vi "Frame_to_word_15693.vi"() -> ()   [LabVIEW 2019]
uses:
  <vilib>/addons/Modulation/Analog/support/mod_Set Error Source.vi
  <vilib>/addons/Modulation/Digital/Support/Common/Validators/mod_Generate Filter Coefficients Validate.vi
  <vilib>/addons/Modulation/Digital/General/subVIs/mod_Generate Filter Coefficients.vi
  <vilib>/addons/Modulation/Digital/General/MT Generate ASK system parameters (M).vi
  <vilib>/addons/Modulation/Analog/MT Modulate AM (DSB).vi
  <vilib>/addons/Modulation/Analog/MT Upconvert Baseband (Real).vi
  <vilib>/measure/macond.llb/IIR Filter for 1 Chan.vi
  <vilib>/express/express analysis/Spectral/Block/exnSpectralBlock spectral measurements RMS poly.vi
  <vilib>/express/express analysis/Spectral/Block/exnSpectralBlock spectral measurements RMS WFM.vi
  <vilib>/addons/Modulation/Analog/MT Downconvert Passband (Real).vi
  <vilib>/addons/Modulation/Analog/MT Demodulate AM (DSB).vi
  <vilib>/ErrorRing/Error Ring.xnode
  <vilib>/express/express analysis/Spectral/XNode/ExpressSpectralMeasurementsBlockNode.xnode
  <vilib>/addons/Modulation/niAMT.lvlib
  <vilib>/measure/NI_MAPro.lvlib
  <vilib>/addons/Modulation/niDMT.lvlib
panel:
  out "lo(x)":u8 format="%x"
  out "hi(x)":u8 format="%x"
  out "DEMODulate 2":cluster{"t0":dbl, "dt":dbl, "Y":dbl[]}(graph)
  out "Array of byte":u8[](array[numeric]) format="%x"
  out "decode":cluster{"t0":dbl, "dt":dbl, "Y":dbl[]}(graph)
  out "Command":cluster{"t0":dbl, "dt":dbl, "Y":dbl[]}(graph)
  out "DEMODulate":cluster{"t0":dbl, "dt":dbl, "Y":dbl[]}(graph)
  out "spectrum analog signal 6":waveform(dbl)(graph)
  out "spectrum analog signal 5":cluster{"t0":dbl, "dt":dbl, "Y":dbl[]}(graph)
  out "Analog signal 8":waveform(dbl)(graph)
  out "spectrum analog signal 4":cluster{"t0":dbl, "dt":dbl, "Y":dbl[]}(graph)
  out "antenna":waveform(dbl)(graph)
  out "summ":waveform(dbl)(graph)
  out "antenna 2":waveform(dbl)(graph)
  out "spectrum analog signal 3":cluster{"t0":dbl, "dt":dbl, "Y":dbl[]}(graph)
  out "spectrum analog signal 2":cluster{"t0":dbl, "dt":dbl, "Y":dbl[]}(graph)
  out "spectrum analog signal":cluster{"t0":dbl, "dt":dbl, "Y":dbl[]}(graph)
  out "SOF+DATA+EOF 2":cluster{"t0":dbl, "dt":dbl, "Y":dbl[]}(graph)
  in  "Value":u8[](array[numeric])=[50] format="%x"
  in  "Mask lenght":u8[](array[numeric])=[119] format="%x"
  in  "AFI":u8[](array[numeric])=[47] format="%x"
  in  "Inventory":u8[](array[numeric])=[161] format="%x"
  out "SOF+DATA+EOF":cluster{"t0":dbl, "dt":dbl, "Y":dbl[]}(graph)
  out "Video":cluster{"t0":dbl, "dt":dbl, "Y":dbl[]}(graph)
  out "video Miller":cluster{"t0":dbl, "dt":dbl, "Y":dbl[]}(graph)
  in  "CARRIER (hz)":dbl
  in  "BIT RATE":dbl
  out "100% ASK":waveform(dbl)(graph)
  in  "Flag":u8[](array[numeric])=[38] format="%x"
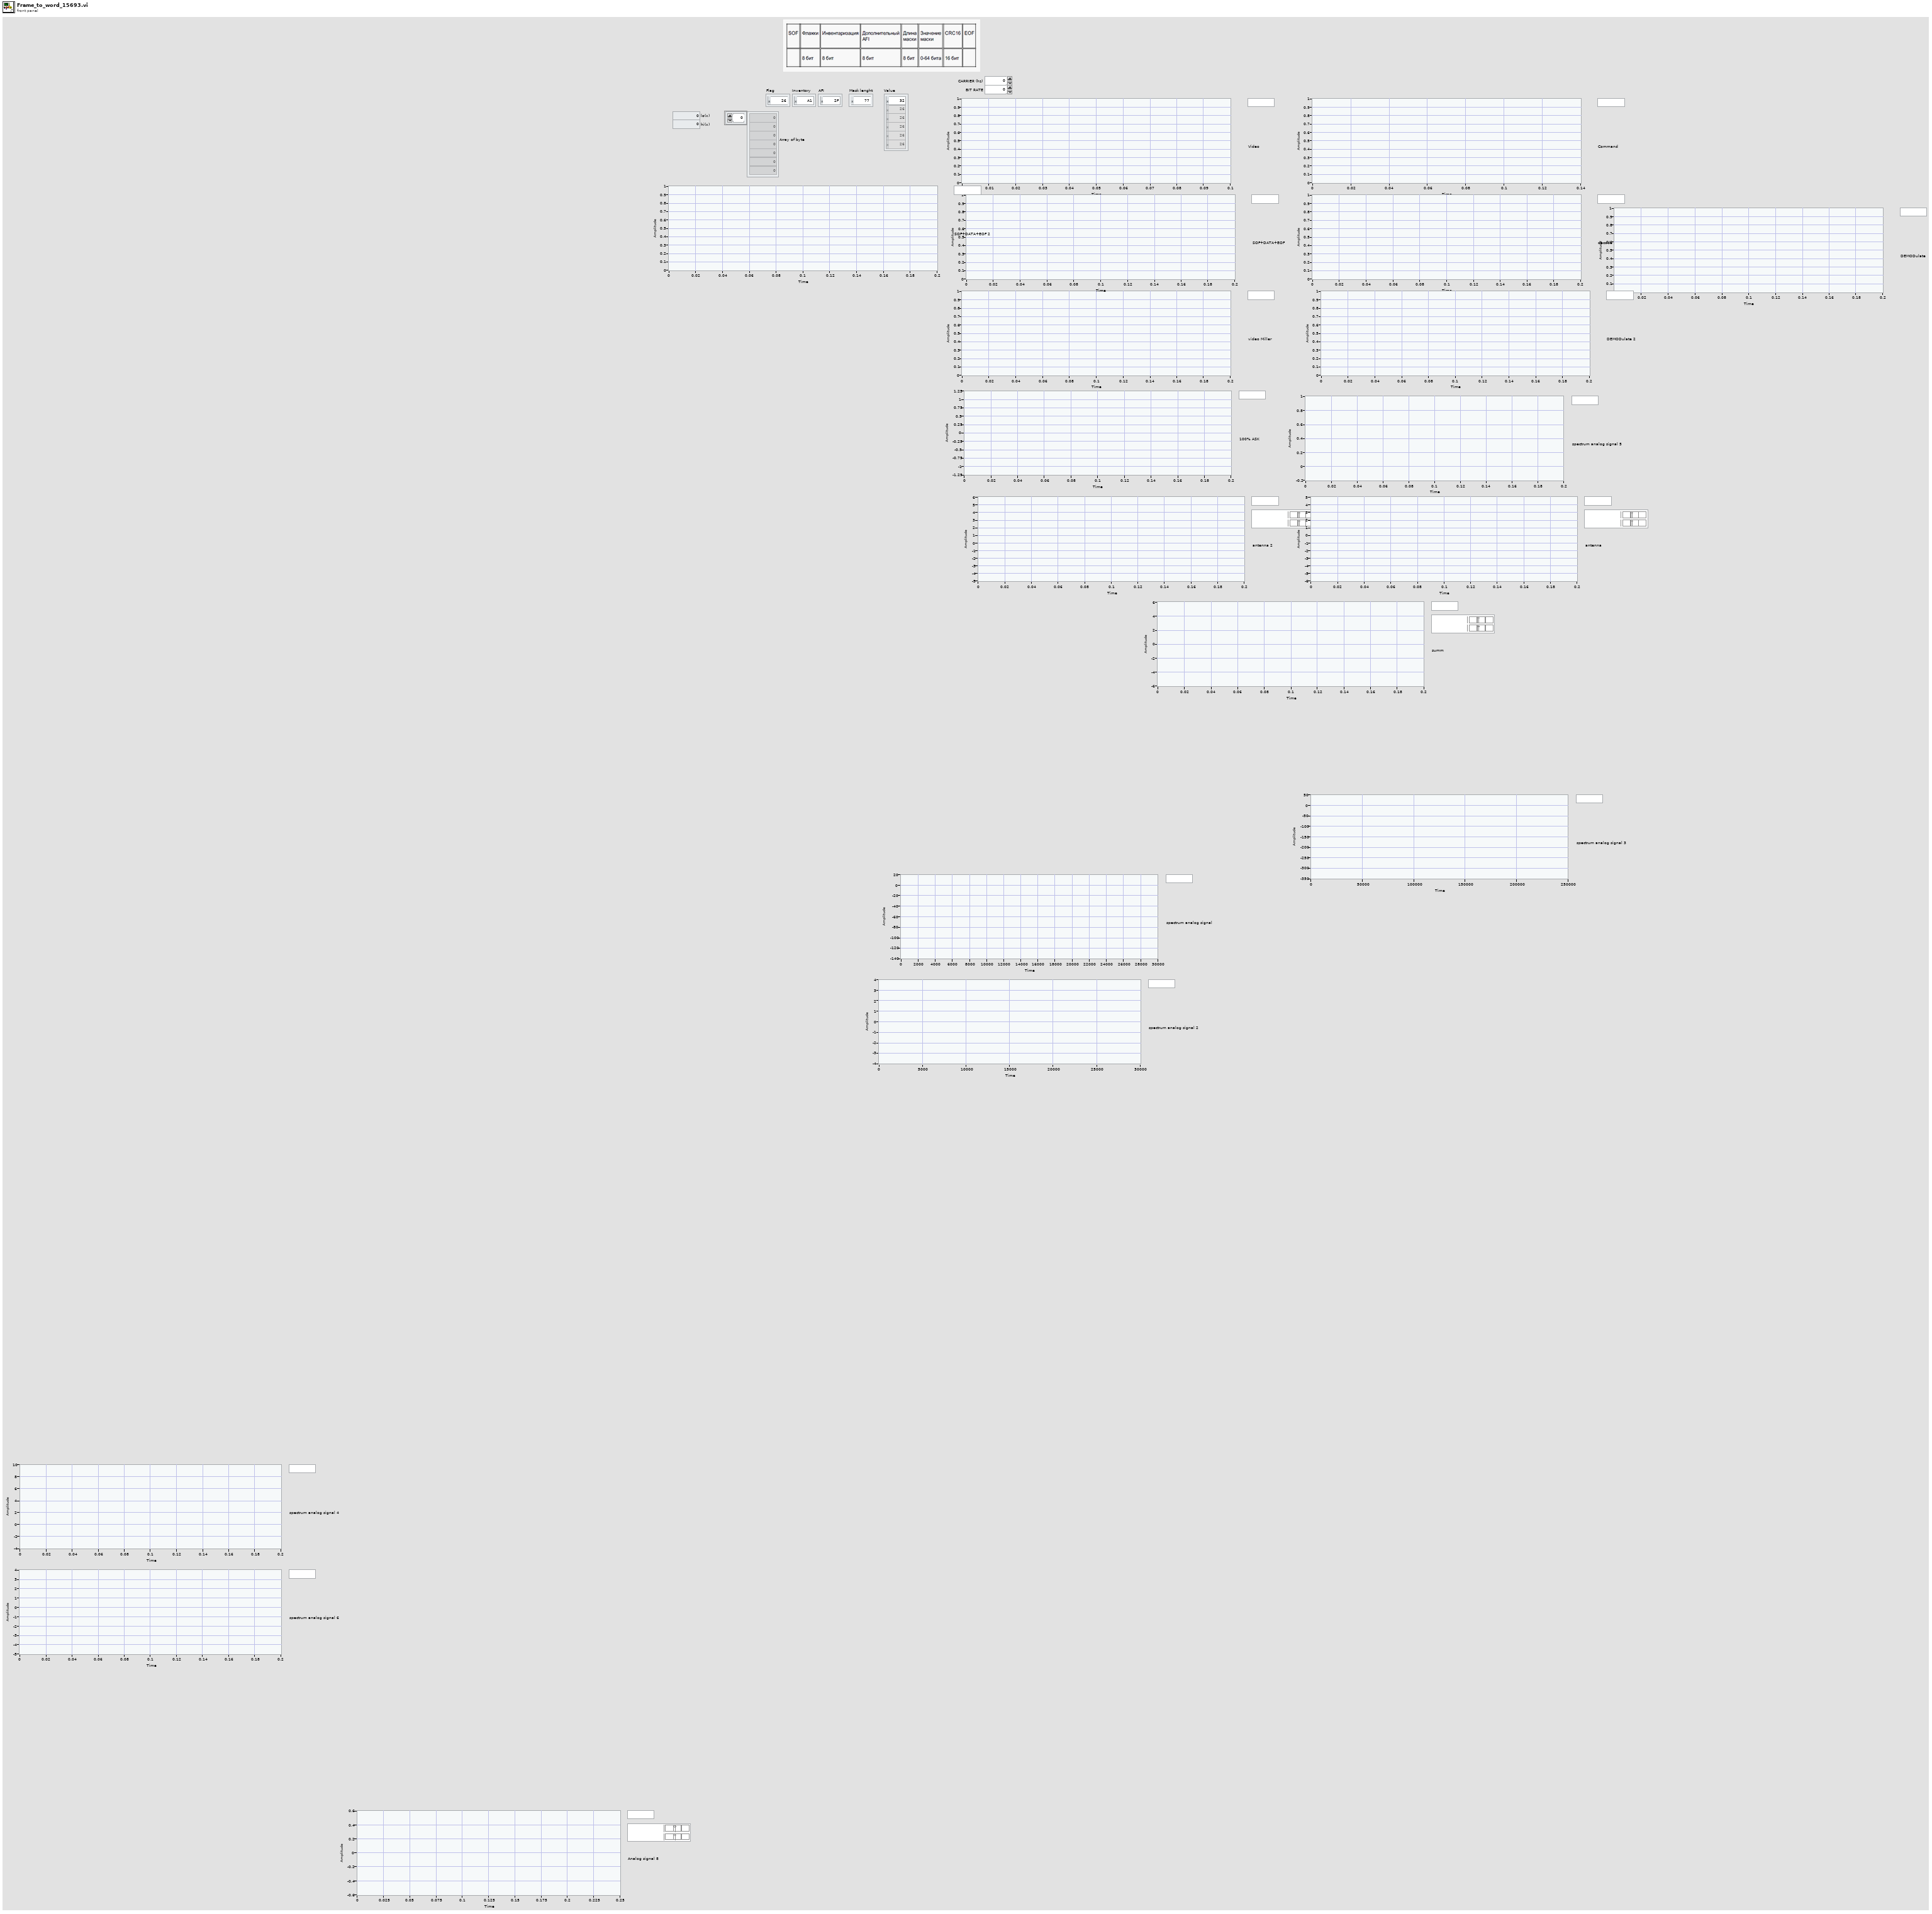
[diagram p1: front panel]
types:
  T1 = enum16{"none", "Raised Cosine", "Root Raised Cos", "Gaussian"}
  T2 = enum16{"FSK", "PSK", "QAM", "MSK", "PAM", "ASK", "CPM"}
  T3 = cluster{"Topology":enum16{"Off", "Butterworth", "Chebyshev", "Inverse Chebyshev", "Elliptic", "Bessel"}, "Type":enum16{"Lowpass", "Highpass", "Bandpass", "Bandstop"}, "Order":i32, "Lower Fc":dbl, "Upper Fc":dbl, "PB Ripple":dbl, "SB Attenuation":dbl}
  T4 = cluster{"passband ripple (dB)":dbl, "stopband start (Hz)":dbl, "stopband gain (dB)":dbl, "compute filter stopband ? (T)":bool}
  T5 = typedef "niAMT.lvlib/Complex Data Waveform.ctl" = cluster{"t0":dbl, "dt":dbl, "Y":cdb[]}
  T6 = cluster{"samples per symbol (16)":i32, "symbol map":cdb[]}
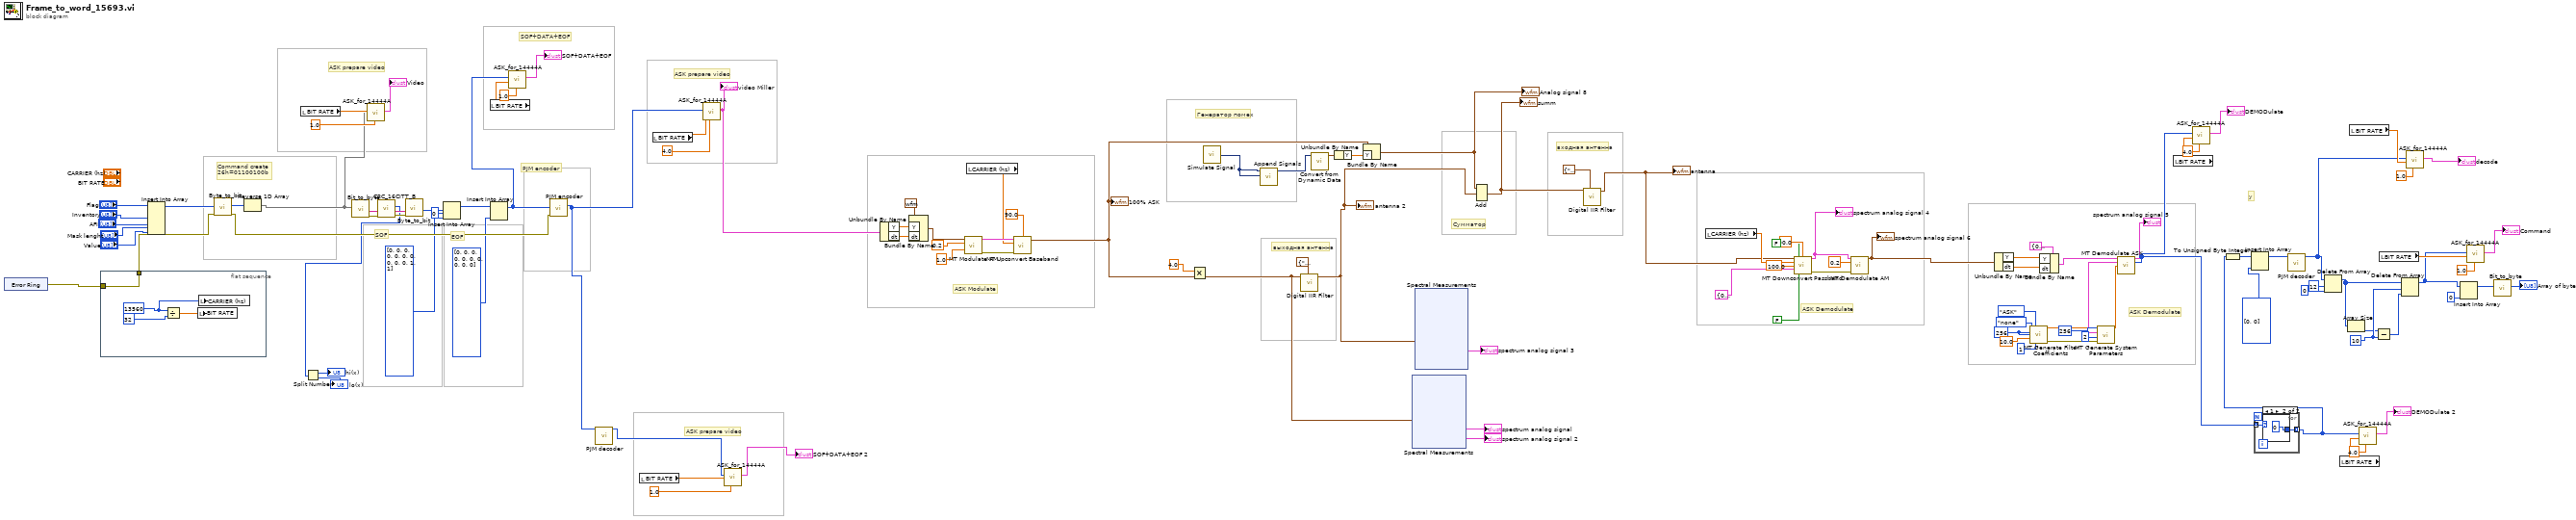
[diagram p0: block diagram]
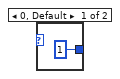
[diagram p2: hidden frame]
diagram:
  w32 = 10 ("length")
  w62 = 256 ("pulse shaping samples per symbol (16)")
  # "у"
  # "ASK Demodulate"
  # "ASK Demodulate"
  # "входная антенна"
  # "Сумматор"
  # "выходная антенна"
  # "Генератор помех"
  # "EOF"
  # "SOF"
  # "ASK prepare video"
  # "ASK Modulate"
  # "SOF+DATA+EOF"
  # "ASK prepare video"
  # "ASK prepare video"
  # "PJM encoder"
  # "Command create \n26h=01100100b"
  n1 = xnode "Error Ring"() -> ("error out"=w99:errorcluster)
  n2 = flat-sequence {
    tunnel: w99 -> [w118]
    tunnel: [w118] -> w98
    frame #0 {
      w119 = u32 13560
      n3 = Divide(x=w119, y=u32 32) -> (x/y=w120:dbl)
      n4 = local write "BIT RATE"(w120) -> ()
      n5 = local write "CARRIER (hz)"(w119) -> ()
    }
  }
  n6 = Insert Into Array(array="Flag", new element #1="Inventory", new element #2="AFI", new element #3="Mask lenght", new element #4="Value") -> (w91:u8[])  [unwired: 1 in]
  n7 = call "Byte_to_bit.vi"("Error In"=w98, "Array of byte"=w91) -> ("Error Out"=w90:errorcluster, "Arrray of bit"=w117:u8[])  [unwired: 5 in, 1 out]
  n8 = Reverse 1D Array(array=w117) -> (reversed array=w9:u8[])
  n9 = local read "BIT RATE"() -> (w107:dbl)
  n10 = call "Bit_to_byte.vi"("Array of bit"=w9) -> ("Error Out"=w7:errorcluster, "BYTE"=w8:string)  [unwired: 8 in, 1 out]
  n11 = call "ASK_for_14444A.vi"("encoder divider"=1.0 ("y"), "BIT RATE"=w107, "Bit stream out (NRZ encode)"=w9) -> ("output complex waveform"=→"Video":T5)  [unwired: 7 in, 1 out]
  n12 = call "CRC_16CITT_B.vi"("Error In"=w7, "DATA PACKET"=w8) -> ("Error Out"=w4:errorcluster, "DATA PACKET+CRC"=w6:string, "CRC out"=w1:u16)  [unwired: 5 in]
  n13 = Split Number(x=w1) -> (hi(x)=→"hi(x)":u8, lo(x)=→"lo(x)":u8)
  n14 = call "Byte_to_bit.vi"("Error In"=w4, "BYTE"=w6) -> ("Arrray of bit (str)"=w5:u8[])  [unwired: 5 in, 2 out]
  n15 = Insert Into Array(array=w5, index=0, new element=u8[] [0, 0, 0, 0, 0, 0, 0, 0, 0, 0, 1, 1] ("Bit stream out (NRZ encode)")) -> (w83:u8[])
  n16 = local read "BIT RATE"() -> (w104:dbl)
  n17 = Insert Into Array(array=w83, new element=u8[] [0, 0, 0, 0, 0, 0, 0, 0, 0, 0] ("Bit stream out (NRZ encode)")) -> (w80:u8[])  [unwired: 1 in]
  n18 = call "ASK_for_14444A.vi"("encoder divider"=1.0 ("y"), "BIT RATE"=w104, "Bit stream out (NRZ encode)"=w80) -> ("output complex waveform"=→"SOF+DATA+EOF":T5)  [unwired: 7 in, 1 out]
  n19 = call "PJM encoder.vi"("Error In"=w90, "Bit stream in"=w80) -> ("Bit stream out (1 from 4)"=w89:u8[])  [unwired: 8 in, 1 out]
  n20 = call "PJM decoder.vi"("Bit stream in"=w89) -> ("output array"=w86:u8[])  [unwired: 9 in, 1 out]
  n21 = local read "BIT RATE"() -> (w87:dbl)
  n22 = local read "BIT RATE"() -> (w116:dbl)
  n23 = call "ASK_for_14444A.vi"("encoder divider"=4.0 ("y"), "BIT RATE"=w116, "Bit stream out (NRZ encode)"=w89) -> ("output complex waveform"=w81:T5)  [unwired: 7 in, 1 out]
  "video Miller" <- w81
  n24 = call "ASK_for_14444A.vi"("encoder divider"=1.0 ("y"), "BIT RATE"=w87, "Bit stream out (NRZ encode)"=w86) -> ("output complex waveform"=→"SOF+DATA+EOF 2":T5)  [unwired: 7 in, 1 out]
  n25 = Unbundle By Name(w81) -> ("Y"=w101:cdb[], "dt"=w100:dbl)
  n26 = Bundle By Name(cluster=waveform(cdb) {"t0"=timestamp(0 s since 1904-01-01), "dt"=1.0, "Y"=[]} ("waveform"), "Y"=w101, "dt"=w100) -> (w110:waveform(cdb))
  n27 = call-poly <vilib>:"MT Modulate AM.vi"("message signal"=w110, "modulation index"=0.2, "peak message amplitude"=1.0) -> ("AM modulated waveform"=w109:cluster{"t0":dbl, "dt":dbl, "Y":cdb[]}, "error out"=w112:errorcluster)  [unwired: 11 in]
  n28 = local read "CARRIER (hz)"() -> (w108:dbl)
  n29 = call-poly <vilib>:"MT Upconvert Baseband.vi"("baseband waveform (complex)"=w109, "initial phase (deg)"=90.0, "carrier frequency (Hz)"=w108, "error in (no error)"=w112) -> ("passband waveform"=w19:waveform(dbl))  [unwired: 10 in, 1 out]
  "100% ASK" <- w19
  n30 = Multiply(x=4.0, y=w19) -> (x*y=w21:waveform(dbl))
  n31 = call "Simulate Signal"() -> ("Sine with Gaussian Noise"=w16:dynamicdata)  [unwired: 14 in, 1 out]
  n32 = call "Append Signals"("Input Signal B"=w16, "Input Signal A"=w16) -> ("Appended Signals"=w15:dynamicdata)  [unwired: 8 in, 1 out]
  n33 = call-poly <vilib>:"Digital IIR Filter.vi"("IIR filter specifications"=T3 {"Topology"=enum."Butterworth", "Type"=enum."Bandpass", "Order"=3, "Lower Fc"=2000.0, "Upper Fc"=22000.0, "PB Ripple"=1.0, "SB Attenuation"=60.0}, "signal in"=w21) -> ("signal out"=w67:waveform(dbl))  [unwired: 7 in, 2 out]
  "antenna 2" <- w67
  n34 = call "Convert from Dynamic Data"("Dynamic Data Type"=w15) -> ("Waveform"=w74:waveform(dbl))  [unwired: 3 in]
  n35 = Unbundle By Name(w74) -> ("Y"=w73:dbl[])
  n36 = Bundle By Name(cluster=w19, "Y"=w73) -> (w66:waveform(dbl))
  "Analog signal 8" <- w66
  n37 = xnode "Spectral Measurements"("Signals"=w21) -> ("FFT - (RMS)"=→"spectrum analog signal":cluster{"f0":dbl, "df":dbl, "magnitude":dbl[]}, "Phase"=→"spectrum analog signal 2":cluster{"f0":dbl, "df":dbl, "phase":dbl[]})  [unwired: 1 in, 1 out]
  n38 = xnode "Spectral Measurements"("Signals"=w67) -> ("FFT - (RMS)"=→"spectrum analog signal 3":cluster{"f0":dbl, "df":dbl, "magnitude":dbl[]})  [unwired: 1 in, 2 out]
  n39 = Add(1:w67, 2:w66) -> (0:w71:waveform(dbl))  [unwired: 1 in, 1 out]
  "summ" <- w71
  n40 = call-poly <vilib>:"Digital IIR Filter.vi"("IIR filter specifications"=T3 {"Topology"=enum."Butterworth", "Type"=enum."Bandpass", "Order"=3, "Lower Fc"=2000.0, "Upper Fc"=22000.0, "PB Ripple"=1.0, "SB Attenuation"=60.0}, "signal in"=w71) -> ("signal out"=w49:waveform(dbl))  [unwired: 7 in, 2 out]
  "antenna" <- w49
  n41 = local read "CARRIER (hz)"() -> (w70:dbl)
  n42 = call-poly <vilib>:"MT Downconvert Passband.vi"("Waveform"=w49, "reset? (F)"=FALSE, "initial phase (deg)"=90.0, "carrier frequency (Hz)"=w70, "passband bandwidth (Hz)"=100.0, "advanced filter parameters"=T4 {"passband ripple (dB)"=0.01, "stopband start (Hz)"=0.0, "stopband gain (dB)"=-96.0, "compute filter stopband ? (T)"=TRUE}, "enable filter (T)"=FALSE) -> ("downconverted waveform (complex baseband)"=w44:T5, "error out"=w50:errorcluster)  [unwired: 5 in, 2 out]
  "spectrum analog signal 4" <- w44
  n43 = call-poly <vilib>:"MT Demodulate AM.vi"("AM modulated waveform"=w44, "modulation index"=0.2, "error in (no error)"=w50) -> ("AM demodulated waveform"=w48:waveform(dbl))  [unwired: 10 in, 2 out]
  "spectrum analog signal 6" <- w48
  n44 = Unbundle By Name(w48) -> ("Y"=w46:dbl[], "dt"=w45:dbl)
  n45 = call <vilib>:"MT Generate Filter Coefficients.vi"("pulse shaping filter (none)"=T1."none", "modulation type"=T2."ASK", "pulse shaping samples per symbol (16)"=w62, "matched samples per symbol (16)"=w62, "filter parameter"=10.0, "filter length (symbols)"=1) -> ("pulse shaping filter coefficients"=w56:dbl[], "error out"=w59:errorcluster)  [unwired: 1 in, 7 out]
  n46 = Bundle By Name(cluster=cluster{"t0":dbl, "dt":dbl, "Y":dbl[]} {"t0"=0.0, "dt"=0.0, "Y"=[]} ("AM modulated waveform"), "Y"=w46, "dt"=w45) -> (w43:cluster{"t0":dbl, "dt":dbl, "Y":dbl[]})
  n47 = call-poly <vilib>:"MT Generate System Parameters.vi"("samples per symbol (16)"=256, "M-ASK (2)"=2, "error in (no error)"=w59) -> ("ASK system parameters"=w57:T6)  [unwired: 12 out]
  n48 = call <vilib>:"MT Demodulate ASK.vi"("input complex waveform"=w43, "ASK system parameters"=w57, "matched filter coefficients"=w56) -> ("recovered complex waveform"=→"spectrum analog signal 5":T5, "output bit stream"=w11:i8[])  [unwired: 8 in, 3 out]
  n49 = local read "BIT RATE"() -> (w40:dbl)
  n50 = call "ASK_for_14444A.vi"("encoder divider"=4.0 ("y"), "BIT RATE"=w40, "Bit stream out (NRZ encode)"=w11) -> ("output complex waveform"=→"DEMODulate":T5)  [unwired: 7 in, 1 out]
  n51 = for {
    tunnel: w11 -> [w123] mode=indexing
    tunnel: [w122] -> w10 mode=indexing
    n52 = case shown="1" w123 {
      tunnel: [u8 1 ("index") u8 0 ("index")] -> w122
      frame 0, Default {
      }
      frame 1 {
      }
    }
  }
  n53 = To Unsigned Byte Integer(number=w10) -> (unsigned 8bit integer=w28:u8[])
  n54 = Insert Into Array(array=w28, new element=u8[] [0, 0]) -> (w18:u8[])  [unwired: 1 in]
  n55 = call "PJM decoder.vi"("Bit stream in"=w18) -> ("output array"=w17:u8[])  [unwired: 9 in, 1 out]
  n56 = Delete From Array(array=w17, length=12, index=0) -> (array with subset deleted=w34:u8[])  [unwired: 1 out]
  n57 = local read "BIT RATE"() -> (w14:dbl)
  n58 = Array Size(array=w34) -> (size(s)=w30:i32)
  n59 = local read "BIT RATE"() -> (w39:dbl)
  n60 = call "ASK_for_14444A.vi"("encoder divider"=4.0 ("y"), "BIT RATE"=w14, "Bit stream out (NRZ encode)"=w10) -> ("output complex waveform"=→"DEMODulate 2":T5)  [unwired: 7 in, 1 out]
  n61 = Subtract(x=w30, y=w32) -> (x-y=w31:i32)
  n62 = local read "BIT RATE"() -> (w35:dbl)
  n63 = Delete From Array(array=w34, length=w32, index=w31) -> (array with subset deleted=w25:u8[])  [unwired: 1 out]
  n64 = call "ASK_for_14444A.vi"("encoder divider"=1.0 ("y"), "BIT RATE"=w39, "Bit stream out (NRZ encode)"=w17) -> ("output complex waveform"=→"decode":T5)  [unwired: 7 in, 1 out]
  n65 = Insert Into Array(array=w25, new element=u8 0 ("new element/subarray")) -> (w23:u8[])  [unwired: 1 in]
  n66 = call "ASK_for_14444A.vi"("encoder divider"=1.0 ("y"), "BIT RATE"=w35, "Bit stream out (NRZ encode)"=w25) -> ("output complex waveform"=→"Command":T5)  [unwired: 7 in, 1 out]
  n67 = call "Bit_to_byte.vi"("Array of bit"=w23) -> ("Array of byte"=→"Array of byte":u8[])  [unwired: 8 in, 2 out]
